vi "MSParametersWindow.vi"() -> ()   [LabVIEW 2017]
uses:
  <vilib>/Utility/config.llb/Read Key (Double).vi
  <vilib>/Utility/config.llb/NI_LVConfig.lvlib
panel:
  in  "Clock 2 [kHz] :":dbl
  in  "Clock 1 [kHz] :":dbl
  in  "Minus 2 [kHz] :":dbl
  in  "Plus 2 [kHz] :":dbl
  in  "Minus 1 [kHz] :":dbl
  in  "Plus 1 [kHz] :":dbl
  in  "Quit":bool
  in  "Gate Time :":dbl
  in  "Gate Detuning :":dbl format="%_3g"
  in  "Stark Shift Ion 2 :":dbl format="%_3g"
  in  "Stark Shift Ion 1 :":dbl format="%_3g"
  in  "Lamb-Dicke Parameter :":dbl format="%_3g"
  in  "Rabi Frequency D :":dbl format="%_4g"
  in  "STR Frequency :":dbl
  in  "Number of Loops :":dbl
  in  "COM Frequency :":dbl
  in  "Rabi Frequency RF :":dbl
  in  "FindParams":bool
  in  "LoadConfig":bool
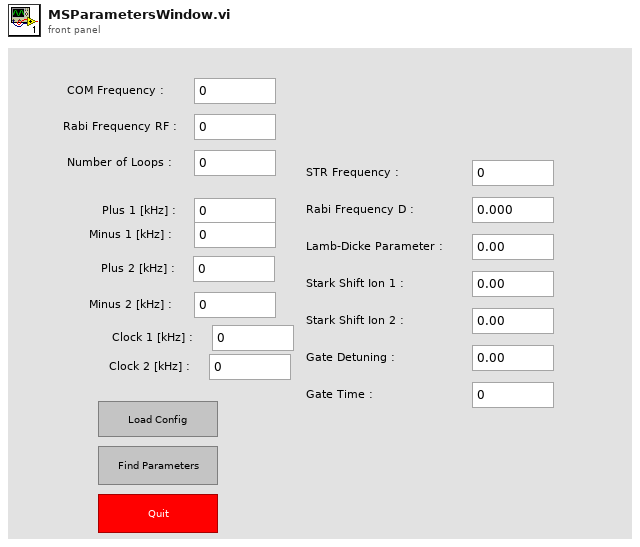
[diagram p1: front panel]
types:
  T1 = typedef "NI_LVConfig.lvlib/Config Data RefNum.ctl" = refnum<k1>
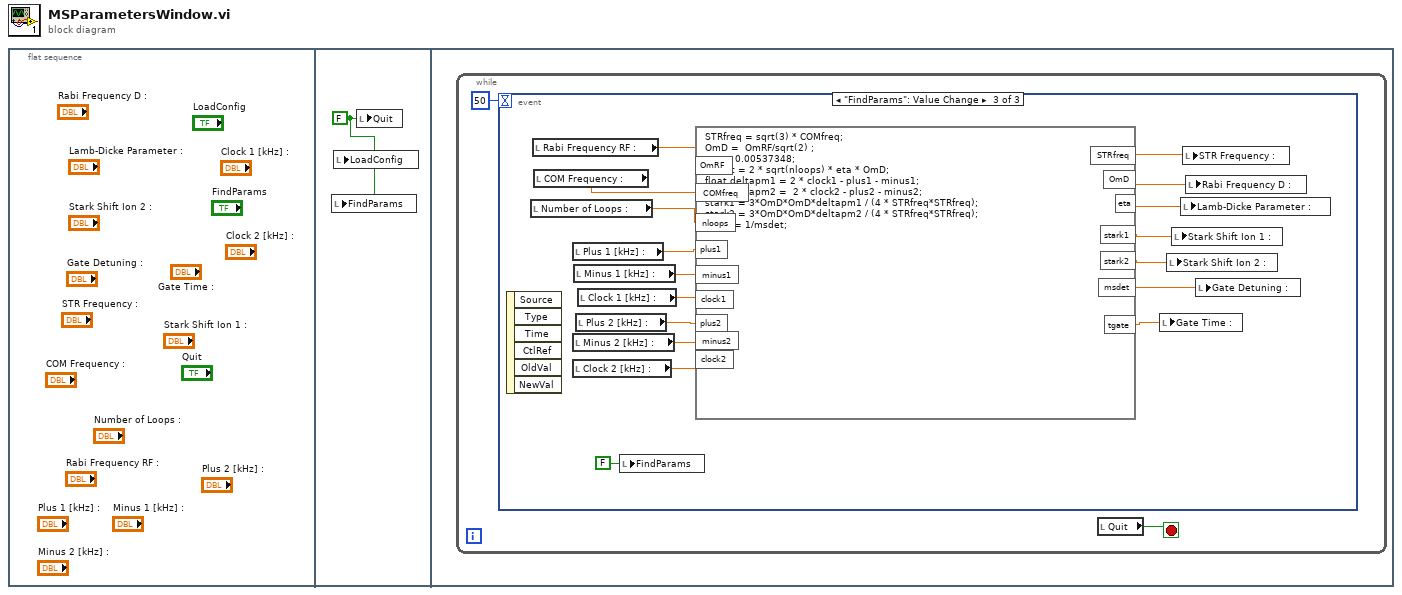
[diagram p0: block diagram]
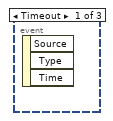
[diagram p2: hidden frame]
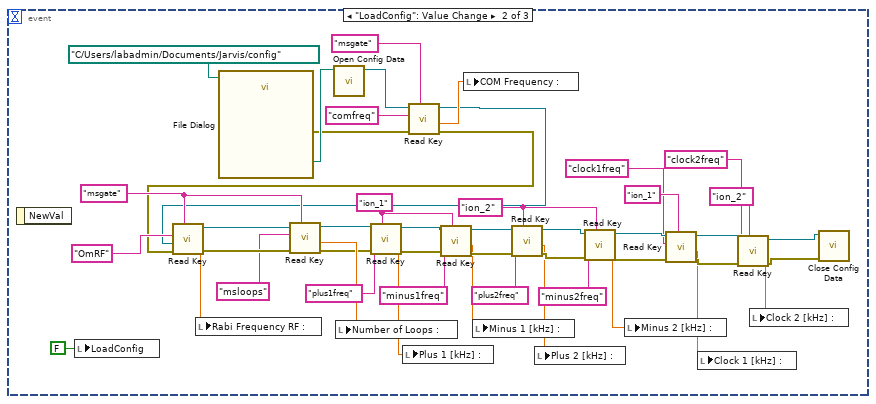
[diagram p3: hidden frame]
diagram:
  n1 = flat-sequence {
    frame #0 {
    }
    frame #1 {
      w1 = FALSE ("Quit")
      n2 = local write "FindParams"(w1) -> ()
      n3 = local write "LoadConfig"(w1) -> ()
      n4 = local write "Quit"(w1) -> ()
    }
    frame #2 {
      n5 = while {
        stop <- w2 stop-if-true
        n6 = event shown="[2] \"FindParams\": Value Change" {
          selector: _ -> [_ _ _]
          dyn-events: _ -> [_ _ _]
          timeout: 50 -> [_ _ _]
          event Timeout {
            n7 = event-data() -> ()  [unwired: 1 in, 3 out]
          }
          event "LoadConfig": Value Change {
            w22 = "ion_2" ("section")
            w25 = "ion_1" ("section")
            w39 = "msgate" ("section")
            n8 = event-data() -> ()  [unwired: 1 in, 1 out]
            n9 = local write "LoadConfig"(FALSE ("LoadConfig")) -> ()
            n10 = call "File Dialog"("start path"=path "C:/Users/labadmin/Documents/Jarvis/config") -> ("selected path"=w50:path, "error out"=w44:errorcluster)  [unwired: 11 in, 2 out]
            n11 = call <vilib>:"Open Config Data.vi"("configuration file path"=w50) -> ("refnum"=w48:T1)  [unwired: 8 in, 2 out]
            n12 = call-poly <vilib>:"Read Key.vi"("section"="msgate", "error in (no error)"=w44, "key"="comfreq", "refnum"=w48) -> ("error out"=w35:errorcluster, "value"=w45:dbl, "refnum out"=w36:T1)  [unwired: 4 in, 1 out]
            n13 = call-poly <vilib>:"Read Key.vi"("section"=w39, "error in (no error)"=w35, "key"="OmRF", "refnum"=w36) -> ("error out"=w40:errorcluster, "value"=w42:dbl, "refnum out"=w41:T1)  [unwired: 4 in, 1 out]
            n14 = local write "Rabi Frequency RF :"(w42) -> ()
            n15 = call-poly <vilib>:"Read Key.vi"("section"=w39, "error in (no error)"=w40, "key"="msloops", "refnum"=w41) -> ("error out"=w29:errorcluster, "value"=w37:dbl, "refnum out"=w33:T1)  [unwired: 4 in, 1 out]
            n16 = local write "Number of Loops :"(w37) -> ()
            n17 = call-poly <vilib>:"Read Key.vi"("section"=w25, "error in (no error)"=w29, "key"="plus1freq", "refnum"=w33) -> ("error out"=w28:errorcluster, "value"=w19:dbl, "refnum out"=w32:T1)  [unwired: 4 in, 1 out]
            n18 = local write "Plus 1 [kHz] :"(w19) -> ()
            n19 = call-poly <vilib>:"Read Key.vi"("section"=w25, "error in (no error)"=w28, "key"="minus1freq", "refnum"=w32) -> ("error out"=w27:errorcluster, "value"=w18:dbl, "refnum out"=w31:T1)  [unwired: 4 in, 1 out]
            n20 = local write "COM Frequency :"(w45) -> ()
            n21 = local write "Minus 1 [kHz] :"(w18) -> ()
            n22 = call-poly <vilib>:"Read Key.vi"("section"=w22, "error in (no error)"=w27, "key"="plus2freq", "refnum"=w31) -> ("error out"=w26:errorcluster, "value"=w17:dbl, "refnum out"=w30:T1)  [unwired: 4 in, 1 out]
            n23 = local write "Plus 2 [kHz] :"(w17) -> ()
            n24 = call-poly <vilib>:"Read Key.vi"("section"=w22, "error in (no error)"=w26, "key"="minus2freq", "refnum"=w30) -> ("error out"=w11:errorcluster, "value"=w16:dbl, "refnum out"=w10:T1)  [unwired: 4 in, 1 out]
            n25 = local write "Minus 2 [kHz] :"(w16) -> ()
            n26 = call-poly <vilib>:"Read Key.vi"("section"="ion_1", "error in (no error)"=w11, "key"="clock1freq", "refnum"=w10) -> ("error out"=w12:errorcluster, "value"=w5:dbl, "refnum out"=w15:T1)  [unwired: 4 in, 1 out]
            n27 = local write "Clock 1 [kHz] :"(w5) -> ()
            n28 = call-poly <vilib>:"Read Key.vi"("section"="ion_2", "error in (no error)"=w12, "key"="clock2freq", "refnum"=w15) -> ("error out"=w13:errorcluster, "value"=w4:dbl, "refnum out"=w14:T1)  [unwired: 4 in, 1 out]
            n29 = local write "Clock 2 [kHz] :"(w4) -> ()
            n30 = call <vilib>:"Close Config Data.vi"("error in (no error)"=w13, "refnum"=w14) -> ()  [unwired: 8 in, 2 out]
          }
          event "FindParams": Value Change {
            n31 = event-data() -> ()  [unwired: 1 in, 6 out]
            n32 = local read "Number of Loops :"() -> (w64:dbl)
            n33 = local read "Rabi Frequency RF :"() -> (w66:dbl)
            n34 = local read "COM Frequency :"() -> (w65:dbl)
            n35 = local read "Plus 1 [kHz] :"() -> (w57:dbl)
            n36 = local read "Minus 2 [kHz] :"() -> (w53:dbl)
            n37 = local read "Clock 2 [kHz] :"() -> (w52:dbl)
            n38 = local read "Minus 1 [kHz] :"() -> (w56:dbl)
            n39 = local read "Plus 2 [kHz] :"() -> (w55:dbl)
            n40 = local read "Clock 1 [kHz] :"() -> (w54:dbl)
            n41 = local write "FindParams"(FALSE ("LoadConfig")) -> ()
            n42 = formula code="STRfreq = sqrt(3) * COMfreq;\nOmD =  OmRF/sqrt(2) ;\neta = 0.00537348;\nmsdet = 2 * sqrt(nloops) * eta * OmD;\nfloat deltapm1 = 2 * clock1 - plus1 - minus1;\nfloat deltapm2 =  2 * clock2 - plus2 - minus2;\nstark1 = 3*OmD*OmD*deltapm1 / (4 * STRfreq*STRfreq); \nstark2 = 3*OmD*OmD*deltapm2 / (4 * STRfreq*STRfreq); \ntgate = 1/msdet;"("OmRF"=w66, "COMfreq"=w65, "nloops"=w64, "plus1"=w57, "minus1"=w56, "clock1"=w54, "plus2"=w55, "minus2"=w53, "clock2"=w52) -> ("OmD"=w61:dbl, "eta"=w62:dbl, "stark1"=w59:dbl, "stark2"=w58:dbl, "msdet"=w60:dbl, "STRfreq"=w63:dbl, "tgate"=w51:dbl)
            n43 = local write "Gate Time :"(w51) -> ()
            n44 = local write "Stark Shift Ion 2 :"(w58) -> ()
            n45 = local write "Stark Shift Ion 1 :"(w59) -> ()
            n46 = local write "Lamb-Dicke Parameter :"(w62) -> ()
            n47 = local write "STR Frequency :"(w63) -> ()
            n48 = local write "Rabi Frequency D :"(w61) -> ()
            n49 = local write "Gate Detuning :"(w60) -> ()
          }
        }
        n50 = local read "Quit"() -> (w2:bool)
      }
    }
  }
